vi "Error.vi"(1 "Weight":dbl[][](array[numeric]), 2 "Forward Error":dbl[](array[numeric]), 3 "Output":dbl[](array[numeric])) -> (0 "Out Error":dbl[](array[numeric]))   [LabVIEW 2009]
uses:
  <vilib>/Analysis/Matrix/Numeric/Conversions/Matrix To Array - RM.vi
  <vilib>/Analysis/Matrix/Numeric/Multiply/Multiply - RM,RM.vi
  <vilib>/Analysis/Matrix/Numeric/Conversions/Array To Matrix - RA2.vi
  <vilib>/Analysis/Matrix/Numeric/Conversions/Array To Matrix - RA.vi
  <vilib>/Analysis/Matrix/NI_Matrix.lvlib
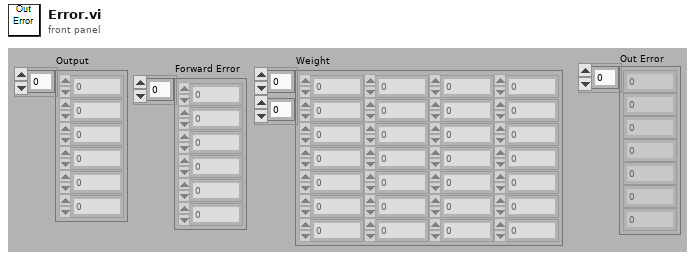
[diagram p1: front panel]
types:
  T1 = typedef "NI_Matrix.lvlib/RealMatrix.ctl" = dbl[][]
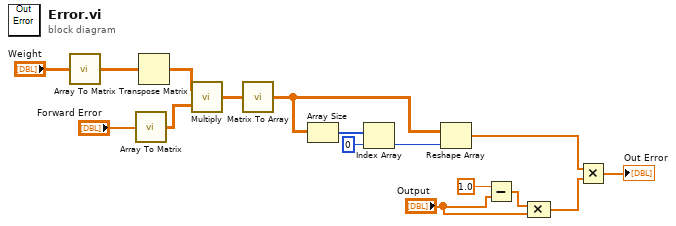
[diagram p0: block diagram]
diagram:
  n1 = call-poly <vilib>:"Array To Matrix.vi"("Real 2D Array"="Weight") -> ("Real Matrix"=w13:T1)
  n2 = call-poly <vilib>:"Array To Matrix.vi"("Real 1D Array"="Forward Error") -> ("Real Matrix (Column Vector)"=w10:T1)
  n3 = Transpose Matrix(1:w13) -> (0:w11:T1)
  n4 = call-poly <vilib>:"Multiply.vi"("Real Matrix B"=w10, "Real Matrix A"=w11) -> ("A * B"=w9:T1)
  n5 = call-poly <vilib>:"Matrix To Array.vi"("Real Matrix"=w9) -> ("Real 2D Array"=w2:dbl[][])
  n6 = Array Size(array=w2) -> (size(s)=w8:i32[])
  n7 = Index Array(array=w8, index=0) -> (element=w6:i32)
  n8 = Reshape Array(w2, w6) -> (w1:dbl[])
  n9 = Subtract(x=1.0, y="Output") -> (x-y=w15:dbl[])
  n10 = Compound Arithmetic op=MULTIPLY(w15, "Output") -> (w5:dbl[])
  n11 = Multiply(x=w1, y=w5) -> (x*y=→"Out Error":dbl[])
